vi "Add Topic.vi"(8 "error in (no error)":errorcluster, 9 "Topic Enqueuer":refnum<class "Message Enqueuer.lvclass">, 10 "Topic Object":refnum<class "Topic.lvclass">, 11 "TopicLookupTable in":refnum<class "TopicLookupTable.lvclass">) -> (0 "error out":errorcluster, 2 "Topic Replaced?":bool, 3 "TopicLookupTable out":refnum<class "TopicLookupTable.lvclass">)   [LabVIEW 2015, in "Mediator.lvlib" / "TopicLookupTable.lvclass"]
uses:
  TopicLookupTable.lvclass
  Topic/Topic.lvclass
  <vilib>/ActorFramework/Message Enqueuer/Message Enqueuer.lvclass
  TopicLookupTable.lvclass/TopicLookupTable.ctl
  Topic/Topic.lvclass/Topic.ctl
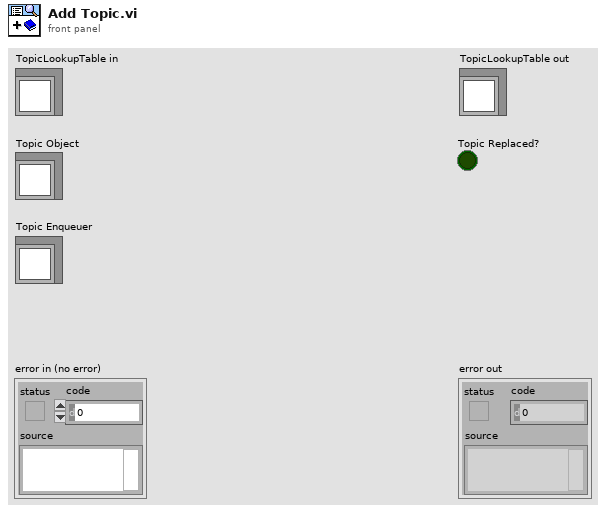
[diagram p1: front panel]
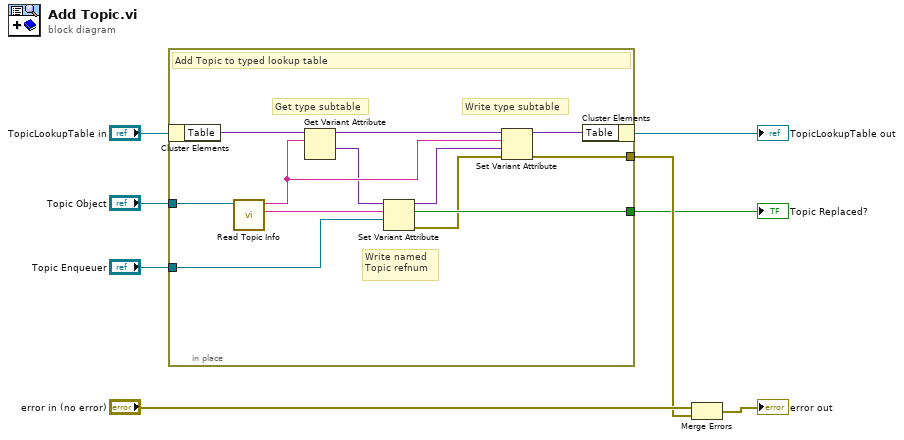
[diagram p0: block diagram]
diagram:
  n1 = in-place {
    in-place-border: [w19] -> w4
    in-place-border: "Topic Object" -> [w10]
    in-place-border: [w12] -> w2
    in-place-border: "Topic Enqueuer" -> [w9]
    # "Write named\nTopic refnum"
    # "Write type subtable"
    # "Get type subtable"
    # "Add Topic to typed lookup table"
    n2 = in-place-cluster #1("TopicLookupTable in") -> ("Table"=w18:variant)
    n3 = call "Read Topic Info.vi"("Topic in"=w10) -> ("Name"=w14:string, "Type"=w15:string)  [unwired: 9 in]
    n4 = Get Variant Attribute(Variant=w18, name=w15) -> (duplicate Variant=w17:variant, value=w13:variant)  [unwired: 2 in, 2 out]
    n5 = Set Variant Attribute(Variant=w13, name=w14, value=w9) -> (Variant out=w16:variant, replaced=w12:bool, error out=w11:errorcluster)  [unwired: 1 in]
    n6 = Set Variant Attribute(Variant=w17, name=w15, value=w16, error in=w11) -> (Variant out=w20:variant, error out=w19:errorcluster)  [unwired: 1 out]
    n7 = in-place-cluster #1("Table"=w20) -> (→"TopicLookupTable out":refnum<class "TopicLookupTable.lvclass">)
  }
  "Topic Replaced?" <- w2
  n8 = Merge Errors("error in (no error)", w4) -> (→"error out":errorcluster)
